vi "Лабораторная №1 Задание 3_8.vi"() -> ()   [LabVIEW 2017]
panel:
  in  "Rmax":dbl
  out "Waveform Chart":dbl(graph)
  out "U вых":dbl
  in  "R вольтметра":dbl
  in  "E":dbl
  in  "R":dbl(slide) scale=0.0..100.0
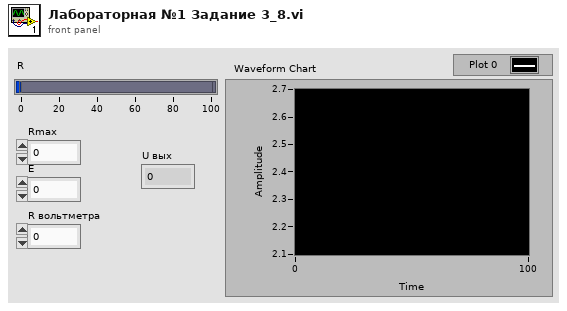
[diagram p1: front panel]
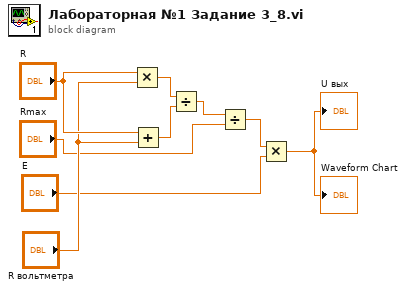
[diagram p0: block diagram]
diagram:
  n1 = Multiply(x="R", y="R вольтметра") -> (x*y=w7:dbl)
  n2 = Add(x="R", y="R вольтметра") -> (x+y=w6:dbl)
  n3 = Divide(x=w7, y=w6) -> (x/y=w5:dbl)
  n4 = Divide(x=w5, y="Rmax") -> (x/y=w2:dbl)
  n5 = Multiply(x=w2, y="E") -> (x*y=→"U вых" →"Waveform Chart":dbl)
